vi "plims.vi"(2 "B":dbl, 3 "Cell Limits":T1, 4 "A":dbl) -> (0 "pmin":dbl, 1 "pmax":dbl)   [LabVIEW 2021]
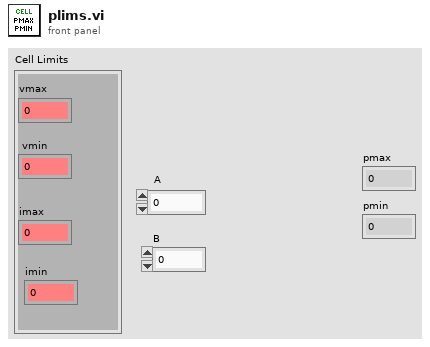
[diagram p1: front panel]
types:
  T1 = cluster{"vmax":dbl, " vmin":dbl, "imax":dbl, "imin":dbl}
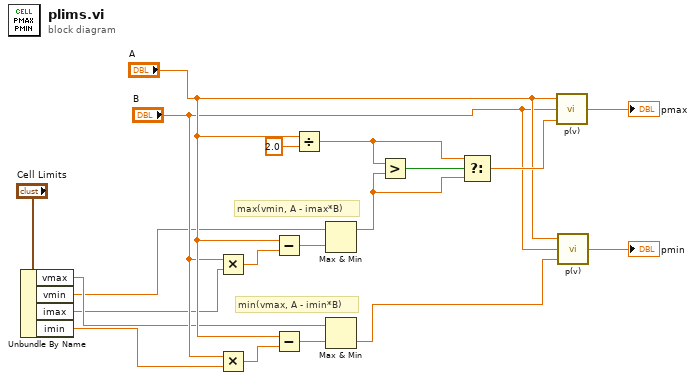
[diagram p0: block diagram]
diagram:
  # "max(vmin, A - imax*B)"
  # "min(vmax, A - imin*B)"
  n1 = Unbundle By Name("Cell Limits") -> ("vmax"=w4:dbl, "vmin"=w2:dbl, "imax"=w1:dbl, "imin"=w3:dbl)
  n2 = Multiply(x="B", y=w1) -> (x*y=w19:dbl)
  n3 = Multiply(x="B", y=w3) -> (x*y=w17:dbl)
  n4 = Subtract(x="A", y=w19) -> (x-y=w18:dbl)
  n5 = Subtract(x="A", y=w17) -> (x-y=w16:dbl)
  n6 = Divide(x="A", y=2.0) -> (x/y=w12:dbl)
  n7 = Max & Min(x=w2, y=w18) -> (max(x,y)=w8:dbl)  [unwired: 1 out]
  n8 = Max & Min(x=w4, y=w16) -> (min(x,y)=w10:dbl)  [unwired: 1 out]
  n9 = Greater?(x=w12, y=w8) -> (0:w13:bool)
  n10 = Select(t=w12, s=w13, f=w8) -> (s? t:f=w11:dbl)
  n11 = call "p(v).vi"("v"=w11, "Z"="B", "E"="A") -> ("p"=→"pmax":dbl)
  n12 = call "p(v).vi"("v"=w10, "Z"="B", "E"="A") -> ("p"=→"pmin":dbl)
